vi "New.vi"(8 "error in (no error)":errorcluster, 11 "reference in":refnum<class "MixedTest TestSuite.lvclass">) -> (0 "error out":errorcluster, 3 "reference out":refnum<class "MixedTest TestSuite.lvclass">)   [LabVIEW 2013, in "MixedTest TestSuite.lvclass"]
uses:
  MixedTest TestSuite.lvclass
  LocationOutsideClassRoot/LocationOutsideClassRoot.lvclass
  Classes/TestCase/TestCase.lvclass
  FrameworkSubTestSuite/FrameworkSubTestSuite.lvclass
  MixedTest TestSuite.lvclass/MixedTest TestSuite.ctl
  Classes/TestSuite/TestSuite.lvclass
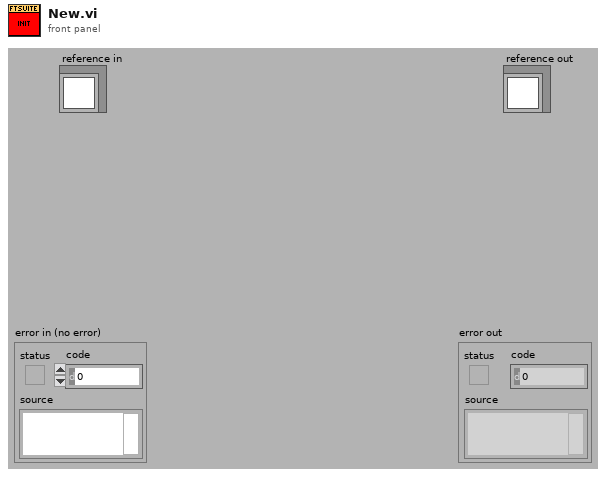
[diagram p1: front panel]
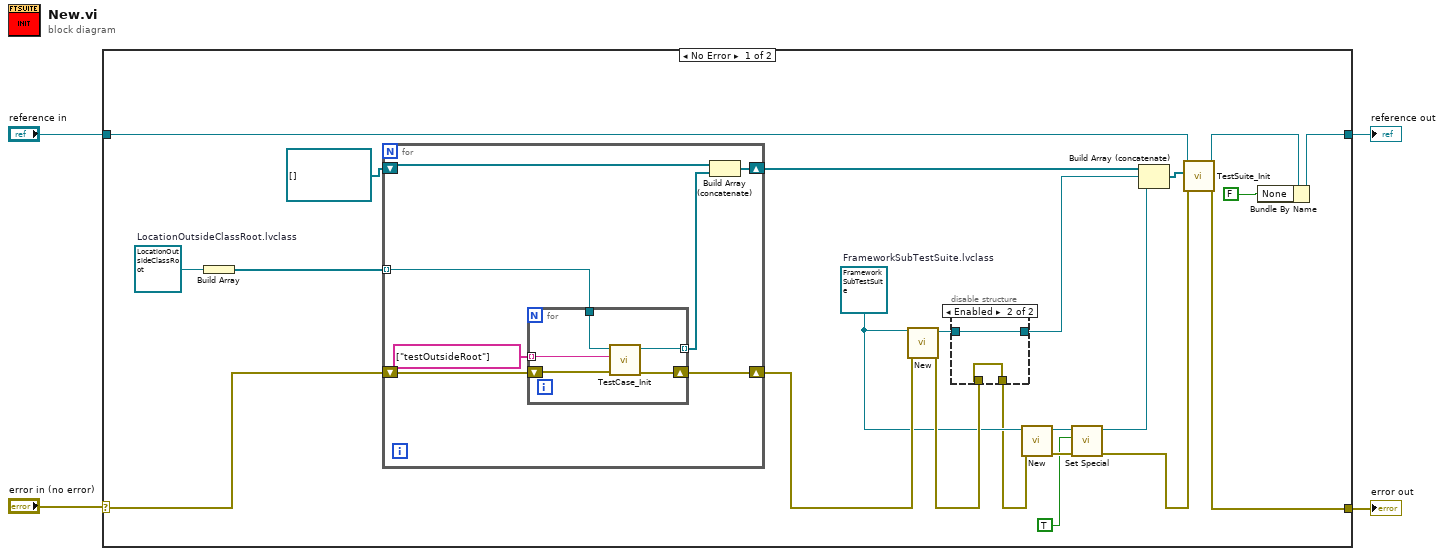
[diagram p0: block diagram]
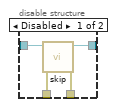
[diagram p2: hidden frame]
diagram:
  n1 = case shown="No Error" "error in (no error)" {
    selector: "error in (no error)" -> [w18 w45]
    tunnel: [w26 w46] -> w4
    tunnel: "reference in" -> [w19 w46]
    tunnel: [w23 w45] -> w1
    frame No Error {
      w11 = refnum<class "FrameworkSubTestSuite.lvclass"> refnum  # FrameworkSubTestSuite.lvclass
      w22 = refnum<class "LocationOutsideClassRoot.lvclass"> refnum  # LocationOutsideClassRoot.lvclass
      n2 = Build Array(w22) -> (w21:refnum<class "LocationOutsideClassRoot.lvclass">[])
      n3 = for {
        shift-right: [w37] -> w15
        shift-left: w18 -> [w38]
        tunnel: w21 -> [w36] mode=indexing
        shift-right: [w33] -> w17
        shift-left: refnum<class "TestCase.lvclass">[] [] -> [w34]
        n4 = for {
          tunnel: w36 -> [w40]
          tunnel: string[] ["testOutsideRoot"] ("tests") -> [w44] mode=indexing
          shift-right: [w42] -> w37
          shift-left: w38 -> [w43]
          tunnel: [w41] -> w35 mode=indexing
          n5 = call "TestCase_Init.vi"("error in (no error)"=w43, "methodName (\"runTest\")"=w44, "TestCase in"=w40) -> ("error out"=w42:errorcluster, "TestCase out"=w41:refnum<class "LocationOutsideClassRoot.lvclass">)  [unwired: 7 in]
        }
        n6 = Build Array (concatenate)(w34, w35) -> (w33:refnum<class "TestCase.lvclass">[])
      }
      n7 = call "New.vi"("error in (no error)"=w15, "reference in"=w11) -> ("error out"=w12:errorcluster, "reference out"=w14:refnum<class "FrameworkSubTestSuite.lvclass">)  [unwired: 8 in]
      n8 = disable-structure shown="Enabled" {
        disable-tunnel: w14 -> [w30 w32]
        disable-tunnel: [w29 w32] -> w13
        disable-tunnel: w12 -> [w28 w31]
        disable-tunnel: [w27 w31] -> w7
        frame Disabled {
          n9 = call "skip.vi"("error in (no error)"=w28, "TestSuite in"=w30) -> ("error out"=w27:errorcluster, "TestSuite out"=w29:refnum<class "FrameworkSubTestSuite.lvclass">)  [unwired: 8 in]
        }
        frame Enabled {
        }
      }
      n10 = call "New.vi"("error in (no error)"=w7, "reference in"=w11) -> ("error out"=w9:errorcluster, "reference out"=w10:refnum<class "FrameworkSubTestSuite.lvclass">)  [unwired: 8 in]
      n11 = call "Set Special.vi"("error in (no error)"=w9, "Special"=TRUE, "FrameworkSubTestSuite in"=w10) -> ("error out"=w8:errorcluster, "FrameworkSubTestSuite out"=w5:refnum<class "FrameworkSubTestSuite.lvclass">)  [unwired: 7 in]
      n12 = Build Array (concatenate)(w17, w13, w5) -> (w16:refnum<class>[])
      n13 = call "TestSuite_Init.vi"("error in (no error)"=w8, "tests (none)"=w16, "TestSuite in"=w19) -> ("error out"=w23:errorcluster, "TestSuite out"=w24:refnum<class "MixedTest TestSuite.lvclass">)  [unwired: 7 in]
      n14 = Bundle By Name(cluster=w24, "None"=FALSE) -> (w26:refnum<class "MixedTest TestSuite.lvclass">)
    }
    frame Error {
    }
  }
  "reference out" <- w4
  "error out" <- w1
